vi "getInstanceEvt.vi"(8 "error in (no error)":errorcluster, 11 "tcpServer in":refnum<class "TcpServer.lvclass">) -> (0 "error out":errorcluster, 1 "EvtWrite":refnum<user-event>, 2 "EvtRead":refnum<user-event>, 3 "tcpServer out":refnum<class "TcpServer.lvclass">)   [LabVIEW 2018, in "TcpServer.lvclass"]
doc: "Get the event user event instances.\n\nEvtRead => receive an event from TCP Client.\nEvtWrite => send an event to TCP Client."
uses:
  TcpServer.lvclass
  TcpServerCmd/typedef/eventTypeDef.ctl
  TcpServerBase/typedef/tcpPacketTypeDef.ctl
  TcpServer.lvclass/TcpServer.ctl
  TcpServerCmd/TcpServerCmd.lvclass/TcpServerCmd.ctl
  TcpServerCmd/TcpServerCmd.lvclass
  TcpServerBase/TcpServerBase.lvclass
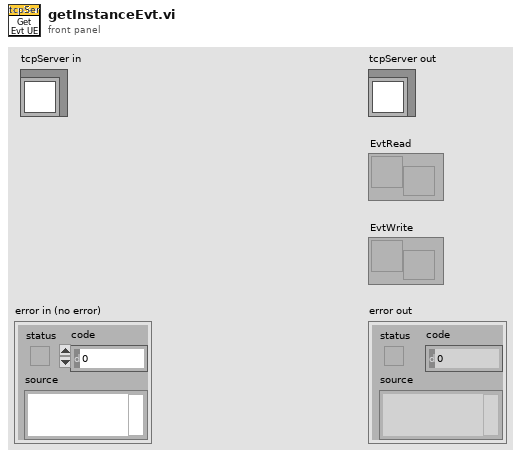
[diagram p1: front panel]
types:
  T1 = typedef "TcpServerCmd.lvclass/userEventTypeDef.ctl" = cluster{"CmdRead":refnum<user-event>, "CmdWrite":refnum<user-event>, "EvtRead":refnum<user-event>, "EvtWrite":refnum<user-event>, "GenRead":refnum<user-event>, "GenWrite":refnum<user-event>}
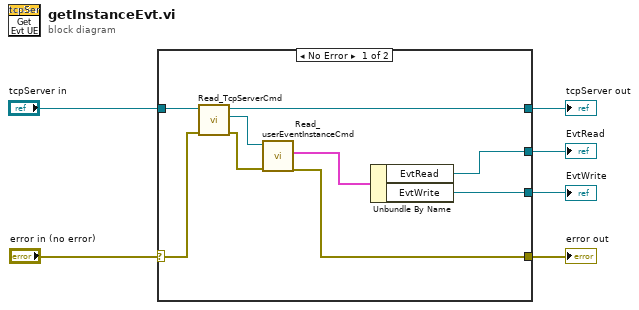
[diagram p0: block diagram]
diagram:
  n1 = case shown="No Error" "error in (no error)" {
    selector: "error in (no error)" -> [w10 w17]
    tunnel: [w13 w17] -> w5
    tunnel: [w8 w16] -> w3
    tunnel: "tcpServer in" -> [w11 w16]
    tunnel: [w14 _] -> w1
    tunnel: [w12 _] -> w2
    frame No Error {
      n2 = call "Read_TcpServerCmd.vi"("error in (no error)"=w10, "TcpServer in"=w11) -> ("error out"=w7:errorcluster, "TcpServerCmd.lvclass"=w9:refnum<class "TcpServerCmd.lvclass">, "TcpServer out"=w8:refnum<class "TcpServer.lvclass">)  [unwired: 7 in]
      n3 = call "Read_userEventInstanceCmd.vi"("error in (no error)"=w7, "TcpServerCmd in"=w9) -> ("error out"=w13:errorcluster, "userEventInstance"=w15:T1)  [unwired: 7 in, 1 out]
      n4 = Unbundle By Name(w15) -> ("EvtRead"=w14:refnum<user-event>, "EvtWrite"=w12:refnum<user-event>)
    }
    frame Error {
    }
  }
  "error out" <- w5
  "tcpServer out" <- w3
  "EvtWrite" <- w2
  "EvtRead" <- w1
